vi "Barcode 1D_Main Function.vi"(0 "Refnum in":T4, 1 "Barcode type strings IN":string[](array[string]), 3 "Number of Matches Requested IN":i32=1 min=1 max=9999, 5 "Barcode Search Options IN":T5, 9 "Barcode Types To Search IN":u32[](array[numeric]), 11 "error in (no error)":errorcluster, 12 "Barcode Grading Options IN":T6, 13 "ROI Descriptor":T1 {"Contours"."Type" items=["No Selection", "Point", "Line", "Rectangle", "Oval", "Polygon", "Free", "Annulus", "Unused2", "Unused3", "Broken Line", "Free Hand Line", "Rotated Rectangle"]}) -> (4 "Refnum out":T4, 6 "Array OUT":cluster{string, string}[](array[cluster]), 10 "Barcode ANSI/CEN/ISO Grading Report OUT":T3(array[cluster]), 14 "Barcodes":T2(array[cluster]) {"Confidence Level" format="%.2f"; "Barcode Type" items=["Reserved", "Codabar", "Code 39", "Code 93", "Code 128", "EAN 8", "EAN 13", "Interleaved 2 of 5", "MSI", "UPCA", "Pharmacode", "RSS Limited"]; "Bounding Box"."y" format="%.2f"; "Bounding Box"."x" format="%.2f"}, 15 "error out":errorcluster)   [LabVIEW 2019]
uses:
  <vilib>/vision/Instrument.llb/Barcode Search Options.ctl
  <vilib>/vision/Image Controls.llb/IMAQ Image.ctl
  <vilib>/vision/NI_Vision_Development_Module.lvlib
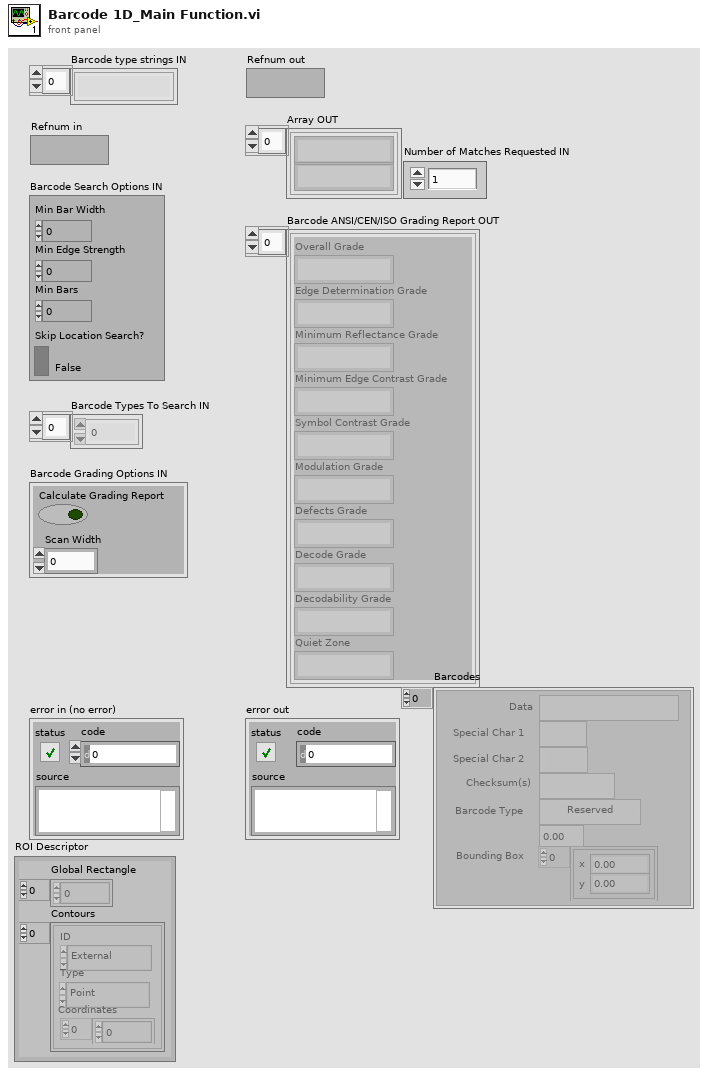
[diagram p1: front panel]
types:
  T1 = cluster{"Global Rectangle":i32[], "Contours":cluster{"ID":enum32{"External", "Internal"}, "Type":u32, "Coordinates":i32[]}[]}
  T2 = cluster{"Data":string, "Special Char 1":string, "Special Char 2":string, "Checksum(s)":string, "Barcode Type":u32, "Confidence Level":sgl, "Bounding Box":cluster{"x":sgl, "y":sgl}[]}[]
  T3 = cluster{"Overall Grade":string, "Edge Determination Grade":string, "Minimum Reflectance Grade":string, "Minimum Edge Contrast Grade":string, "Symbol Contrast Grade":string, "Modulation Grade":string, "Defects Grade":string, "Decode Grade":string, "Decodability Grade":string, "Quiet Zone":string}[]
  T4 = typedef "IMAQ Image.ctl" = refnum<image>
  T5 = typedef "Barcode Search Options.ctl" = cluster{"Min Bar Width":u32, "Min Edge Strength":u32, "Min Bars":u32, "Skip Location Search?":bool}
  T6 = cluster{"Calculate Grading Report":bool, "Scan Width ":i32}
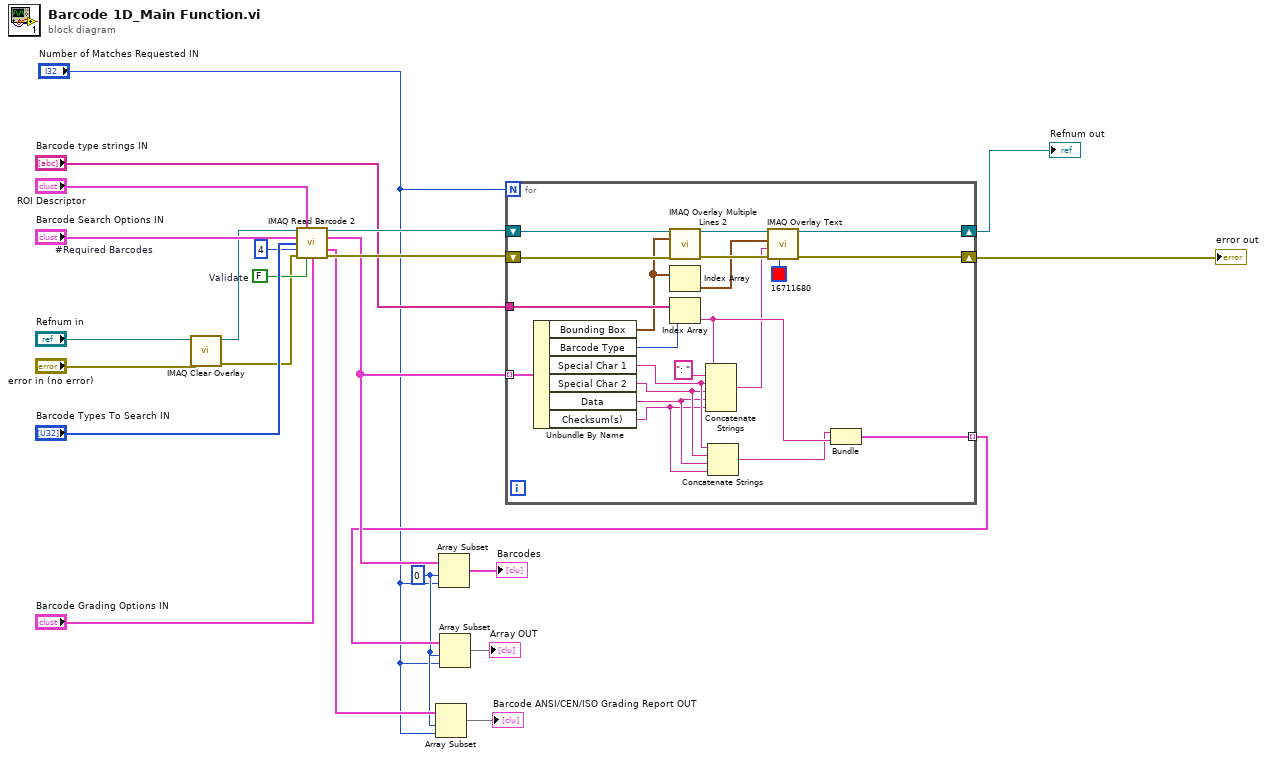
[diagram p0: block diagram]
diagram:
  w2 = 0 ("index")
  w14 = u32 4  # #Required Barcodes
  w18 = FALSE  # Validate
  n1 = call "IMAQ Clear Overlay"("error in (no error)"="error in (no error)", "Image"="Refnum in") -> ("error out"=w10:errorcluster, "Image Out"=w11:T4)  [unwired: 8 in]
  n2 = call "IMAQ Read Barcode 2"("Image"=w11, "ROI Descriptor"="ROI Descriptor", "Barcode Search Options"="Barcode Search Options IN", "Barcode Types To Search"="Barcode Types To Search IN", "Num of Required Barcodes"=w14, "error in (no error)"=w10, "Validate"=w18, "Barcode Grading Options"="Barcode Grading Options IN") -> ("Image (duplicate)"=w16:T4, "Barcodes"=w8:T2, "Barcode ANSI/CEN/ISO Grading Report"=w4:T3, "error out"=w17:errorcluster)  [unwired: 3 in, 1 out]
  n3 = Array Subset(array=w4, index=w2, length="Number of Matches Requested IN") -> (→"Barcode ANSI/CEN/ISO Grading Report OUT":T3)
  n4 = Array Subset(array=w8, index=w2, length="Number of Matches Requested IN") -> (→"Barcodes":T2)
  n5 = for {
    N: "Number of Matches Requested IN" -> [_]
    tunnel: w8 -> [w44] mode=indexing
    tunnel: "Barcode type strings IN" -> [w43]
    shift-right: [w39] -> w19
    shift-left: w16 -> [w35]
    shift-right: [w36] -> w20
    shift-left: w17 -> [w38]
    tunnel: [w32] -> w6 mode=indexing
    n6 = Unbundle By Name(w44) -> ("Bounding Box"=w24:cluster{"x":sgl, "y":sgl}[], "Barcode Type"=w33:u32, "Special Char 1"=w29:string, "Special Char 2"=w28:string, "Data"=w27:string, "Checksum(s)"=w26:string)
    n7 = call "IMAQ Overlay Multiple Lines 2"("Image"=w35, "Line End Points"=w24, "error in (no error)"=w38) -> ("Image Out"=w41:T4, "error out"=w37:errorcluster)  [unwired: 11 in]
    n8 = Index Array(array=w24) -> (element=w34:cluster{"x":sgl, "y":sgl})  [unwired: 1 in]
    n9 = Index Array(array=w43, index=w33) -> (element=w31:string)
    n10 = Concatenate Strings(w31, ": " ("string"), w29, w28, w27, w26) -> (w30:string)
    n11 = Concatenate Strings(w29, w28, w27, w26) -> (w25:string)
    n12 = call "IMAQ Overlay Text"("Text Color (black)"=u32 16711680, "error in (no error)"=w37, "String"=w30, "Origin"=w34, "Image"=w41) -> ("error out"=w36:errorcluster, "Image Out"=w39:T4)  [unwired: 5 in]
    n13 = Bundle(w25, w31) -> (w32:cluster{string, string})  [unwired: 1 in]
  }
  "error out" <- w20
  "Refnum out" <- w19
  n14 = Array Subset(array=w6, index=w2, length="Number of Matches Requested IN") -> (→"Array OUT":cluster{string, string}[])
